vi "test - String with Keywords.vi"(8 "error in (no error)":errorcluster, 11 "TestCase in":refnum<class "testcase-Supported-Datatype.lvclass">) -> (0 "error out":errorcluster, 3 "TestCase out":refnum<class "testcase-Supported-Datatype.lvclass">)   [LabVIEW 2017, in "testcase-Supported-Datatype.lvclass"]
uses:
  testcase-Supported-Datatype.lvclass
  b40cf643-f38a-46f9-a5a3-634c21c9432c.vi
  9f15237e-ebd8-4d7f-a756-ec2da678f0ff.vi
  00d33017-f56b-420e-b77c-1e7c4d83746c.vi
  08aaf221-0d2d-4d3d-9c04-42c4c1c9dd4f.vi
  af7b55ab-96f5-4dfe-9a6e-dcc75dd624d1.vi
  addons/API-String-Arugments-Support/_Support/Convert API String Arguments to Data(variant).vi
  <vilib>/addons/_JKI Toolkits/VI Tester/TestCase.llb/TestCase.lvclass
  C:/Program Files (x86)/National Instruments/LabVIEW 2017/vi.lib/addons/_JKI Toolkits/VI Tester/TestCase.llb/TestCase.lvclass
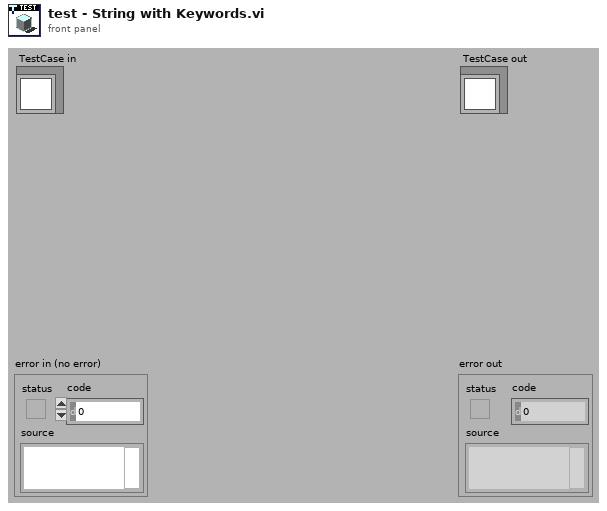
[diagram p1: front panel]
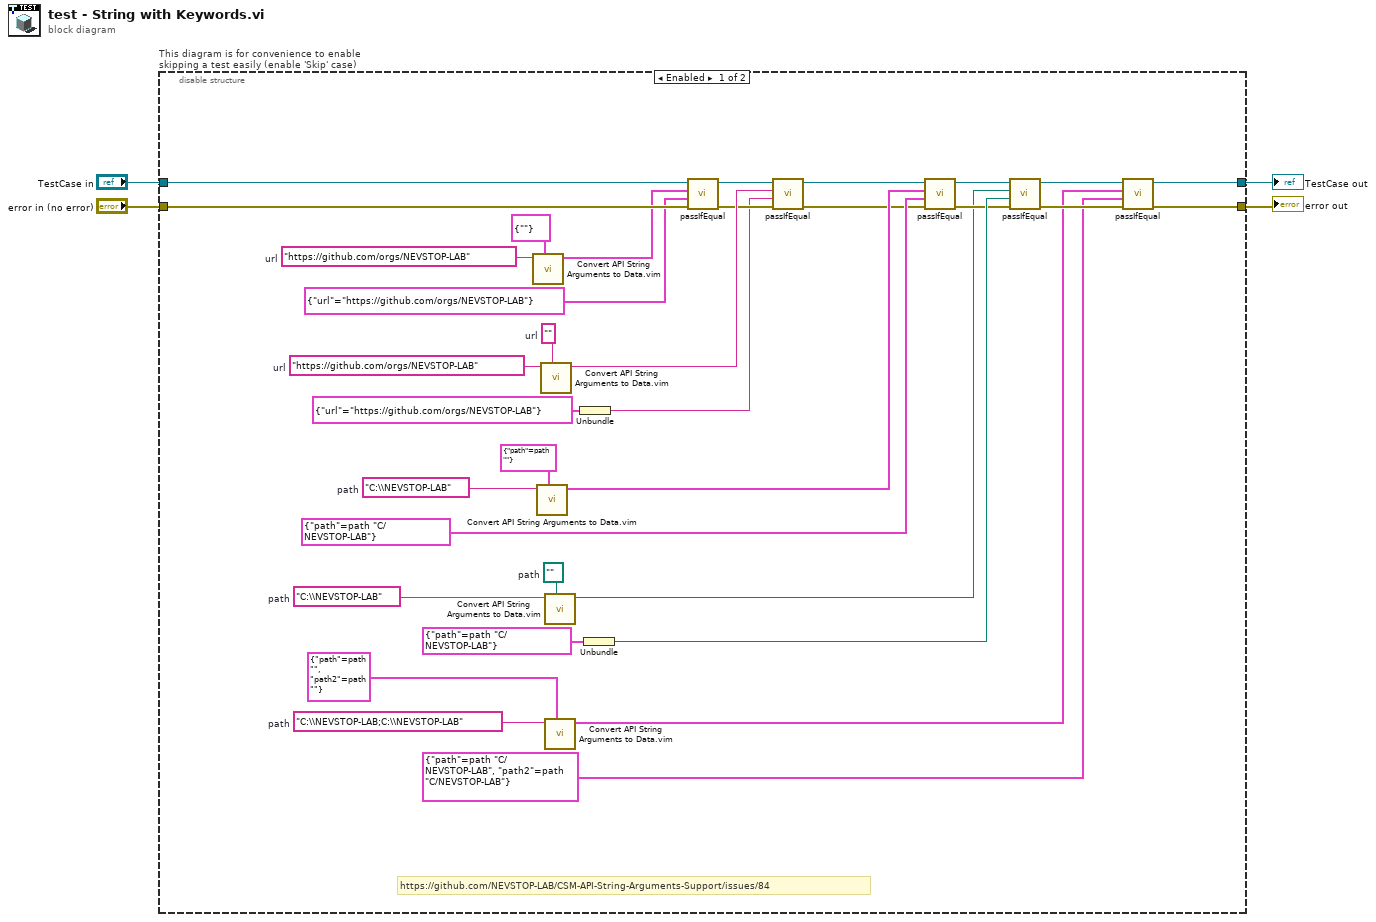
[diagram p0: block diagram]
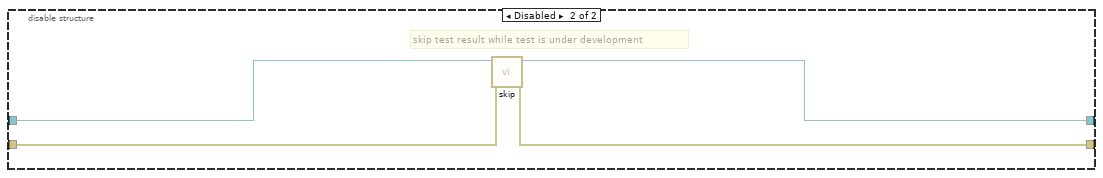
[diagram p2: hidden frame]
diagram:
  n1 = disable-structure "This diagram is for convenience to enable skipping a test easily (enable 'Skip' case)" shown="Enabled" {
    disable-tunnel: "TestCase in" -> [w38 w42]
    disable-tunnel: [w7 w40] -> w1
    disable-tunnel: [w8 w41] -> w3
    disable-tunnel: "error in (no error)" -> [w37 w39]
    frame Enabled {
      w12 = "C:\\NEVSTOP-LAB;C:\\NEVSTOP-LAB"  # path
      w24 = path ""  # path
      w21 = "C:\\NEVSTOP-LAB"  # path
      w16 = "C:\\NEVSTOP-LAB"  # path
      w27 = ""  # url
      w30 = "https://github.com/orgs/NEVSTOP-LAB"  # url
      w35 = "https://github.com/orgs/NEVSTOP-LAB"  # url
      # "https://github.com/NEVSTOP-LAB/CSM-API-String-Arguments-Support/issues/84"
      n2 = call "Convert API String Arguments to Data.vim"("Reference Type"=cluster{"url":string} {"url"=""}, "API String"=w35) -> ("Data"=w34:cluster{"url":string})  [unwired: 6 in, 1 out]
      n3 = call "Convert API String Arguments to Data.vim"("Reference Type"=cluster{"path":path} {"path"=path ""}, "API String"=w16) -> ("Data"=w17:cluster{"path":path})  [unwired: 6 in, 1 out]
      n4 = call "Convert API String Arguments to Data.vim"("Reference Type"=w27, "API String"=w30) -> ("Data"=w31:string)  [unwired: 6 in, 1 out]
      n5 = call "Convert API String Arguments to Data.vim"("Reference Type"=w24, "API String"=w21) -> ("Data"=w20:path)  [unwired: 6 in, 1 out]
      n6 = call "Convert API String Arguments to Data.vim"("Reference Type"=cluster{"path":path, "path2":path} {"path"=path "", "path2"=path ""}, "API String"=w12) -> ("Data"=w6:cluster{"path":path, "path2":path})  [unwired: 6 in, 1 out]
      n7 = Unbundle(cluster{"url":string} {"url"="https://github.com/orgs/NEVSTOP-LAB"}) -> ("url"=w26:string)
      n8 = Unbundle(cluster{"path":path} {"path"=path "C:/NEVSTOP-LAB"}) -> ("path"=w25:path)
      n9 = call-dynamic "passIfEqual.vi"("error in (no error)"=w37, "y"=cluster{"url":string} {"url"="https://github.com/orgs/NEVSTOP-LAB"}, "x"=w34, "TestCase in"=w38) -> ("error out"=w28:errorcluster, "TestCase out"=w29:refnum<class "testcase-Supported-Datatype.lvclass">)  [unwired: 6 in]
      n10 = call-dynamic "passIfEqual.vi"("error in (no error)"=w28, "y"=w26, "x"=w31, "TestCase in"=w29) -> ("error out"=w13:errorcluster, "TestCase out"=w14:refnum<class "testcase-Supported-Datatype.lvclass">)  [unwired: 6 in]
      n11 = call-dynamic "passIfEqual.vi"("error in (no error)"=w13, "y"=cluster{"path":path} {"path"=path "C:/NEVSTOP-LAB"}, "x"=w17, "TestCase in"=w14) -> ("error out"=w23:errorcluster, "TestCase out"=w22:refnum<class "testcase-Supported-Datatype.lvclass">)  [unwired: 6 in]
      n12 = call-dynamic "passIfEqual.vi"("error in (no error)"=w23, "y"=w25, "x"=w20, "TestCase in"=w22) -> ("error out"=w9:errorcluster, "TestCase out"=w10:refnum<class "testcase-Supported-Datatype.lvclass">)  [unwired: 6 in]
      n13 = call-dynamic "passIfEqual.vi"("error in (no error)"=w9, "y"=cluster{"path":path, "path2":path} {"path"=path "C:/NEVSTOP-LAB", "path2"=path "C:/NEVSTOP-LAB"}, "x"=w6, "TestCase in"=w10) -> ("error out"=w8:errorcluster, "TestCase out"=w7:refnum<class "testcase-Supported-Datatype.lvclass">)  [unwired: 6 in]
    }
    frame Disabled {
      # "skip test result while test is under development"
      n14 = call <vilib>:"skip.vi"("error in (no error)"=w39, "TestCase in"=w42) -> ("error out"=w41:errorcluster, "TestCase out"=w40:refnum<class "testcase-Supported-Datatype.lvclass">)  [unwired: 8 in]
    }
  }
  "error out" <- w3
  "TestCase out" <- w1
